vi "Table Stage Module.vi"(8 "Error In":errorcluster) -> (0 "Error Out":errorcluster)   [LabVIEW 2014]
uses:
  Controls/SingleAxisStageCtrls.ctl
  Stage Global Variables.vi
panel:
  out "Axis [Out]":T1
  in  "Axis [In]":T1
  in  "Actions":T2(ring)=enum."Init"
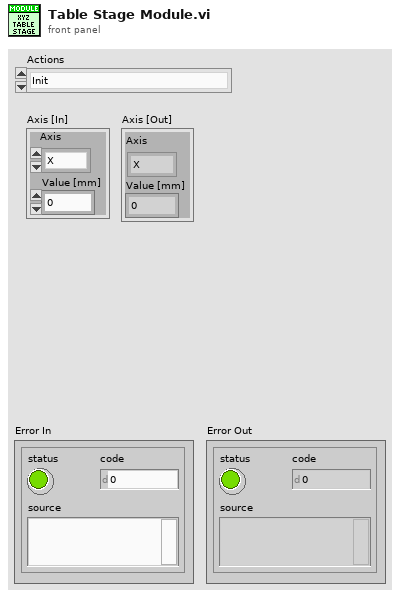
[diagram p1: front panel]
types:
  T1 = typedef "SingleAxisStageCtrls.ctl" = cluster{"Axis":enum16{"X", "Y", "Z"}, "Value [mm]":dbl}
  T2 = enum16{"Unknown", "Init", "Connect", "Step", "Move", "Stop", "Get Position", "Set Limits", "Disconnect"}
  T3 = typedef "TableStageModels.ctl" = enum16{"None", "CONEX-CC"}
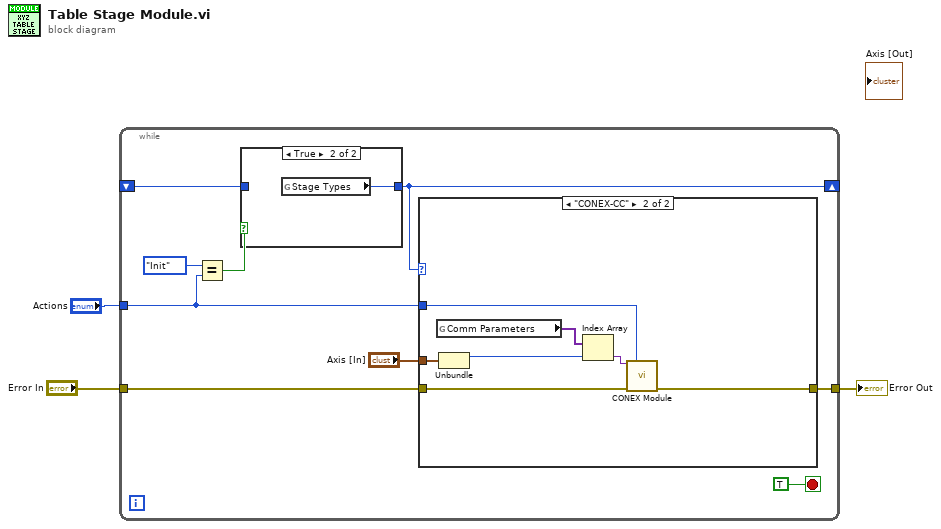
[diagram p0: block diagram]
diagram:
  n1 = while {
    tunnel: "Error In" -> [w11]
    tunnel: [w10] -> w2
    shift-right: [w6] -> _
    shift-left: _ -> [w5]
    tunnel: "Actions" -> [w9]
    stop <- TRUE stop-if-true
    n2 = Equal?(x=T2."Init", y=w9) -> (x = y?=w7:bool)
    n3 = case shown="True" w7 {
      tunnel: [w13 w14] -> w6
      tunnel: w5 -> [w13 _]
      frame False {
      }
      frame True {
        n4 = global read "Stage Global Variables.vi" "Stage Types"() -> (w14:T3)
      }
    }
    n5 = case shown="\"CONEX-CC\"" w6 {
      tunnel: w11 -> [w15 w18]
      tunnel: [w15 w21] -> w10
      tunnel: w9 -> [_ w22]
      tunnel: "Axis [In]" -> [_ w20]
      frame "None", Default {
      }
      frame "CONEX-CC" {
        n6 = global read "Stage Global Variables.vi" "Comm Parameters"() -> (w17:variant[])
        n7 = Unbundle(w20) -> ("Axis"=w19:enum16{"X", "Y", "Z"})  [unwired: 1 out]
        n8 = Index Array(array=w17, index=w19) -> (element=w16:variant)
        n9 = call "CONEX Module.vi"("Device Cfg [In]"=w16, "Actions"=w22, "Error In"=w18) -> ("Error Out"=w21:errorcluster)  [unwired: 8 in, 4 out]
      }
    }
  }
  "Error Out" <- w2
